vi "get..vi"(5 "Stop (F)":bool, 7 "error in":errorcluster) -> (20 "Image Out":T1(plugin-control), 26 "Stopped":bool, 27 "error out":errorcluster)   [LabVIEW 2017]
doc: "Creates, and edits acquisitions using the NI Vision Acquisition Express VI.\n\nThe NI Vision Acquisition Wizard is launched by placing the Express VI on the block diagram. Select an acquisition source and configure an acquisition using NI-IMAQ, NI-IMAQdx, or simulate an acquisition by reading an AVI or image files from a folder. After an acquisition is configured, select controls and indicators to be able to programmatically set in LabVIEW. Double-click the Vision Acquisition Express VI to edit the acquisition.\n\nNote: Any images created by the Express VI need to be disposed after use. Use the IMAQ Dispose.vi to cleanup the images output by the Express VI when they are no longer needed."
uses:
  <vilib>/vision/driver/NI_Vision_Acquisition_Software.lvlib
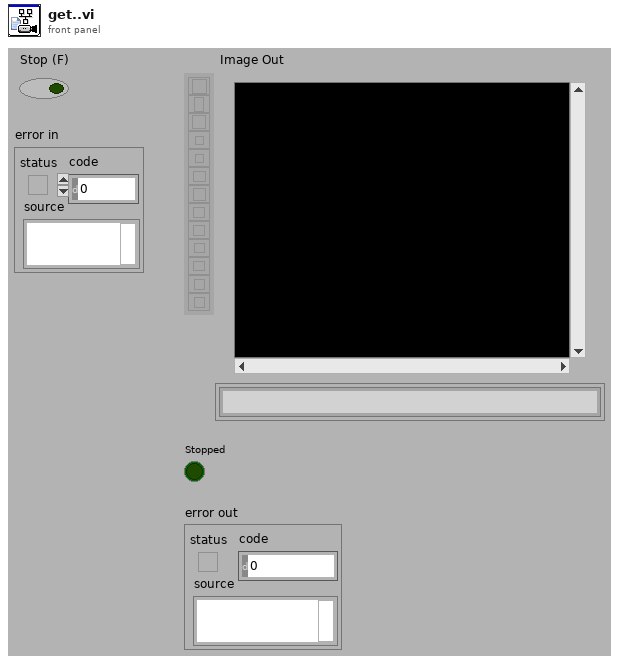
[diagram p1: front panel]
types:
  T1 = typedef "IMAQ Image.ctl" = refnum<image>
  T2 = typedef "IMAQdx.ctl" = refnum<k21>
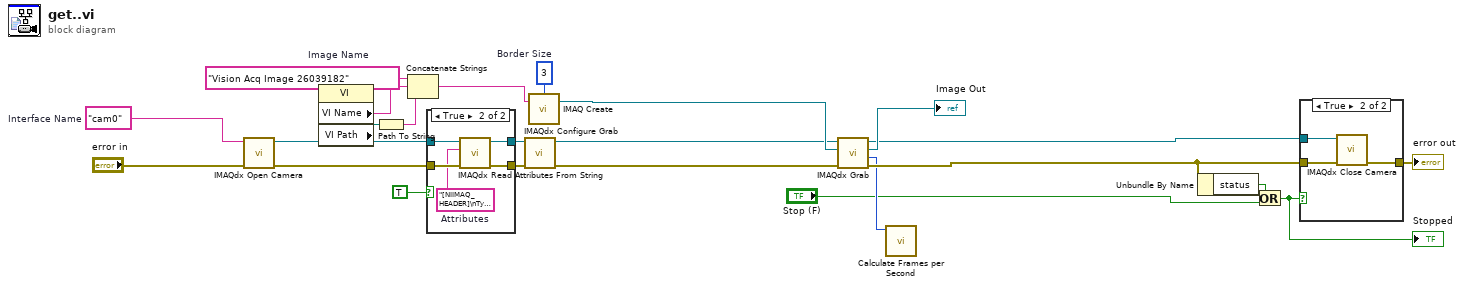
[diagram p0: block diagram]
diagram:
  w1 = 3  # Border Size
  w7 = "Vision Acq Image 26039182"  # Image Name
  w22 = "cam0"  # Interface Name
  n1 = call <vilib>:"IMAQdx Open Camera.vi"("error in"="error in", "Session In"=w22) -> ("error out"=w5:errorcluster, "Session Out"=w6:T2)  [unwired: 1 in, 7 out]
  n2 = property class="VI"() -> ("VI Name"=w10:string, "VI Path"=w11:path)  [unwired: 2 in, 2 out]
  n3 = Path To String(path=w11) -> (string=w9:string)
  n4 = Concatenate Strings(w7, w10, w9) -> (w8:string)
  n5 = case shown="True" TRUE ("Init Attributes") {
    tunnel: w6 -> [w26 w31]
    tunnel: w5 -> [w25 w30]
    tunnel: [w26 w28] -> w4
    tunnel: [w25 w27] -> w3
    frame False {
    }
    frame True {
      w29 = "[NIIMAQ_HEADER]\nType = 2\nVersion = 8\n\n[CAMERA_DATA]\nAcquisitionAttributes::Bayer::Algorithm = \"Bilinear\"\nAcquisitionAttributes::Bayer::GainB = \"1\"\nAcquisitionAttributes::Bayer::GainG = \"1\"\nAcquisitionAttributes::Bayer::GainR = \"1\"\nAcquisitionAttributes::Bayer::Pattern = \"Use hardware value\"\nAcquisitionAttributes::BitsPerPixel = \"Use hardware value\"\nAcquisitionAttributes::IgnoreFirstFrame = \"false\"\nAcquisitionAttributes::ImageDecoderCopyMode = \"Auto\"\nAcquisitionAttributes::OutputImageType = \"Auto\"\nAcquisitionAttributes::OverwriteMode = \"Get Newest\"\nAcquisitionAttributes::PixelSignedness = \"Use hardware value\"\nAcquisitionAttributes::ReceiveTimestampMode = \"None\"\nAcquisitionAttributes::ShiftPixelBits = \"false\"\nAcquisitionAttributes::SwapPixelBytes = \"false\"\nAcquisitionAttributes::Timeout = \"5000\"\nAcquisitionAttributes::VideoMode = \"640 x 480 YUY 2 30.00 fps\"\nCameraAttributes::BacklightCompensation::Mode = \"Manual\"\nCameraAttributes::BacklightCompensation::Value = \"0\"\nCameraAttributes::Brightness::Mode = \"Manual\"\nCameraAttributes::Brightness::Value = \"135\"\nCameraAttributes::Contrast::Mode = \"Manual\"\nCameraAttributes::Contrast::Value = \"5\"\nCameraAttributes::Exposure::Mode = \"AutoAperaturePriority\"\nCameraAttributes::Focus::Mode = \"Manual\"\nCameraAttributes::Focus::Value = \"10\"\nCameraAttributes::Pan::Mode = \"Manual\"\nCameraAttributes::Pan::Value = \"0\"\nCameraAttributes::PowerLineFrequency::Mode = \"60Hz\"\nCameraAttributes::Saturation::Mode = \"Manual\"\nCameraAttributes::Saturation::Value = \"83\"\nCameraAttributes::Sharpness::Mode = \"Manual\"\nCameraAttributes::Sharpness::Value = \"25\"\nCameraAttributes::Tilt::Mode = \"Manual\"\nCameraAttributes::Tilt::Value = \"0\"\nCameraAttributes::WhiteBalance::Mode = \"Auto\"\nCameraAttributes::Zoom::Mode = \"Manual\"\nCameraAttributes::Zoom::Value = \"0\"\n"  # Attributes
      n6 = call <vilib>:"IMAQdx Read Attributes From String.vi"("error in"=w30, "Attributes String In"=w29, "Session In"=w31) -> ("error out"=w27:errorcluster, "Session Out"=w28:T2)  [unwired: 7 out]
    }
  }
  n7 = call <vilib>:"IMAQdx Configure Grab.vi"("error in"=w3, "Session In"=w4) -> ("error out"=w23:errorcluster, "Session Out"=w19:T2)  [unwired: 8 out]
  n8 = call "IMAQ Create"("Border Size"=w1, "Image Name"=w8) -> ("New Image"=w20:T1)  [unwired: 2 in, 2 out]
  n9 = call <vilib>:"IMAQdx Grab.vi"("error in"=w23, "Image In"=w20, "Session In"=w19) -> ("error out"=w18:errorcluster, "Buffer Number Out"=w17:u32, "Image Out"=→"Image Out":T1, "Session Out"=w16:T2)  [unwired: 1 in, 4 out]
  n10 = call <vilib>:"Calculate Frames per Second.vi"("Buffer Number"=w17) -> ()  [unwired: 2 in, 9 out]
  n11 = Unbundle By Name(w18) -> ("status"=w12:bool)
  n12 = Or(x=w12, y="Stop (F)") -> (x .or. y?=w13:bool)
  "Stopped" <- w13
  n13 = case "Case Structure_template1" shown="True" w13 {
    tunnel: [w32 w34] -> w15
    tunnel: w18 -> [w32 w35]
    tunnel: w16 -> [_ w33]
    frame False {
    }
    frame True {
      n14 = call <vilib>:"IMAQdx Close Camera.vi"("error in"=w35, "Session In"=w33) -> ("error out"=w34:errorcluster)  [unwired: 9 out]
    }
  }
  "error out" <- w15
